vi "yaqc_get_position.vi"(8 "error in (no error)":errorcluster, 9 "Yaqc Client In":refnum<k38>, 10 "Python Module Path In":path, 11 "Python Session In":refnum<k35>) -> (0 "error out":errorcluster, 1 "Yaqc Client Out":refnum<k38>, 2 "Python Module Path Out":path, 3 "Python Session Out":refnum<k35>, 4 "position":dbl)   [LabVIEW 2022 SP3]
doc: "Provides the current position for the selected device."
uses:
  <vilib>/Utility/error.llb/Simple Error Handler.vi
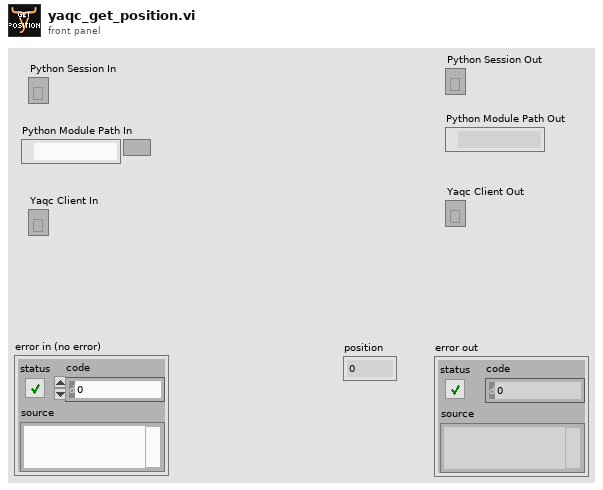
[diagram p1: front panel]
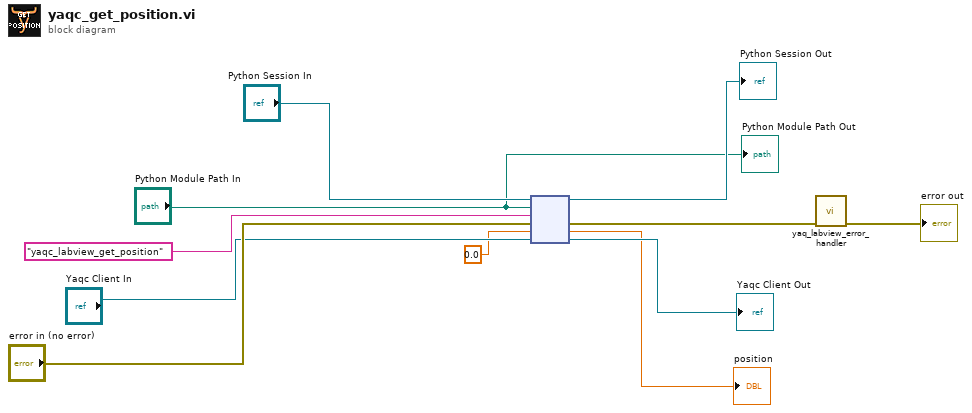
[diagram p0: block diagram]
diagram:
  n1 = node("Python Session In", "Python Module Path In", "yaqc_labview_get_position" ("function name"), "error in (no error)", 0.0, "Yaqc Client In") -> (→"Python Session Out":refnum<k35>, w8:errorcluster, →"position":dbl, →"Yaqc Client Out":refnum<k38>)  [unwired: 2 out]
  n2 = call "yaq_labview_error_handler.vi"("error in (no error)"=w8) -> ("error out"=→"error out":errorcluster)  [unwired: 10 in]
  "Python Module Path Out" <- "Python Module Path In"
